vi "Test.vi"() -> ()   [LabVIEW 2020]
uses:
  <userlib>/lvwamp/WAMP Client/WAMP Client.lvclass
panel:
  in  "Port":u16=8080
  in  "Address":string="localhost"
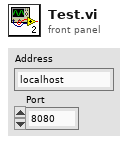
[diagram p1: front panel]
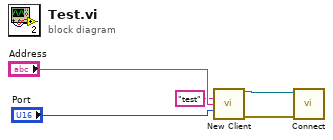
[diagram p0: block diagram]
diagram:
  n1 = call <userlib>:"New Client.vi"("Realm"="test", "Address"="Address", "Port"="Port") -> ("reference out"=w3:refnum<class "WAMP Client.lvclass">, "error out"=w2:errorcluster)  [unwired: 11 in]
  n2 = call <userlib>:"Connect.vi"("error in (no error)"=w2, "WAMP Client in"=w3) -> ()  [unwired: 8 in, 2 out]
